vi "Write Client Certs.vi"(8 "error in (no error)":errorcluster, 10 "Client Certs":T1[](array[typedef]), 11 "dotNET SSL Client Socket in":refnum<class "dotNET SSL Client Socket.lvclass">) -> (0 "error out":errorcluster, 3 "dotNET SSL Client Socket out":refnum<class "dotNET SSL Client Socket.lvclass">)   [LabVIEW 2013, in "dotNET SSL Socket.lvlib" / "dotNET SSL Client Socket.lvclass"]
uses:
  dotNET SSL Client Socket.lvclass
  dotNET SSL Socket/PFX Certificate.ctl
  dotNET SSL Client Socket.lvclass/dotNET SSL Client Socket.ctl
  dotNET SSL Socket/dotNET SSL Socket.lvclass
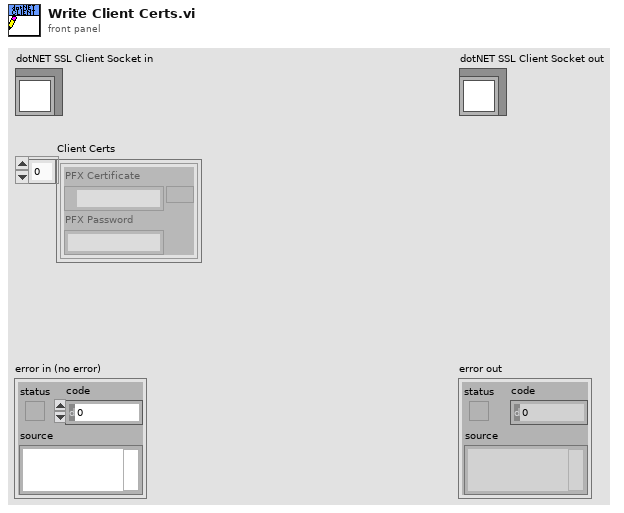
[diagram p1: front panel]
types:
  T1 = typedef "dotNET SSL Socket.lvlib/dotNET SSL Socket.lvclass/PFX Certificate.ctl" = cluster{"PFX Certificate":path, "PFX Password":string}
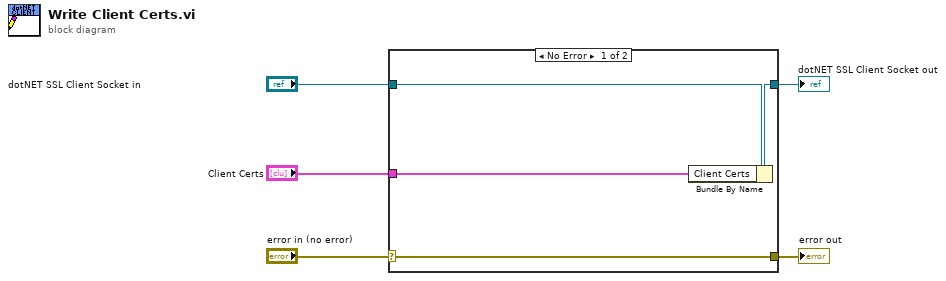
[diagram p0: block diagram]
diagram:
  n1 = case shown="No Error" "error in (no error)" {
    selector: "error in (no error)" -> [w9 w10]
    tunnel: [w9 w10] -> w4
    tunnel: [w7 w11] -> w2
    tunnel: "dotNET SSL Client Socket in" -> [w8 w11]
    tunnel: "Client Certs" -> [w6 _]
    frame No Error {
      n2 = Bundle By Name(cluster=w8, "Client Certs"=w6) -> (w7:refnum<class "dotNET SSL Client Socket.lvclass">)
    }
    frame Error {
    }
  }
  "error out" <- w4
  "dotNET SSL Client Socket out" <- w2
